vi "Host_Save_Datagram.vi"(11 "Path":path) -> ()   [LabVIEW 2018]
uses:
  <vilib>/Utility/file.llb/Write Delimited Spreadsheet (DBL).vi
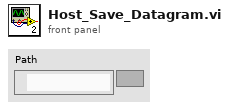
[diagram p1: front panel]
types:
  T1 = cluster{dbl, "Double":dbl, "Double":dbl, "Double":dbl}
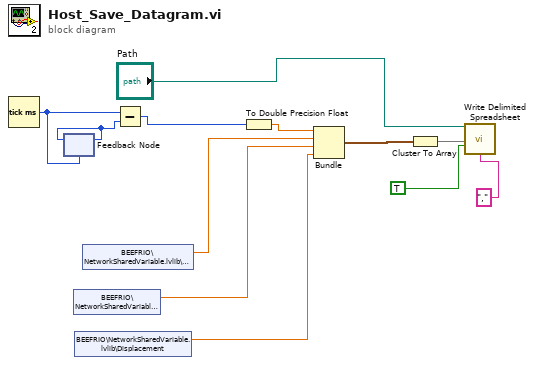
[diagram p0: block diagram]
diagram:
  n1 = Tick Count (ms)() -> (millisecond timer value=w2:u32)
  n2 = feedback #1(w2) -> (w1:u32)
  n3 = feedback-in #1(w1) -> ()
  n4 = shared-variable "BEEFRIO\\NetworkSharedVariable.lvlib\\Velocity"() -> (w5:dbl)  [unwired: 1 in, 1 out]
  n5 = shared-variable "BEEFRIO\\NetworkSharedVariable.lvlib\\Displacement"() -> (w6:dbl)  [unwired: 1 in, 1 out]
  n6 = shared-variable "BEEFRIO\\NetworkSharedVariable.lvlib\\Acceleration"() -> (w7:dbl)  [unwired: 1 in, 1 out]
  n7 = Subtract(x=w2, y=w1) -> (x-y=w3:u32)
  n8 = To Double Precision Float(number=w3) -> (double precision float=w4:dbl)
  n9 = Bundle(w4, "Double"=w7, "Double"=w5, "Double"=w6) -> (w11:T1)  [unwired: 1 in]
  n10 = Cluster To Array(cluster=w11) -> (array=w10:dbl[])
  n11 = call-poly <vilib>:"Write Delimited Spreadsheet.vi"("file path (dialog if empty)"="Path", "1D data"=w10, "append to file? (new file:F)"=TRUE, "delimiter (\\t)"=",") -> ()  [unwired: 10 in, 2 out]
